vi "OpenNewFile.vi"(8 "error in (no error)":errorcluster, 10 "targetFolder":path, 11 "FileAppender in":refnum<class "FileAppender.lvclass">) -> (0 "error out":errorcluster, 3 "FileAppender out":refnum<class "FileAppender.lvclass">)   [LabVIEW 2026, in "Lumberjack.lvlib" / "FileAppender.lvclass"]
uses:
  FileAppender.lvclass
  FileAppender.lvclass/FileAppender.ctl
  Lumberjack.lvlib
  Appender.lvclass/Appender.lvclass
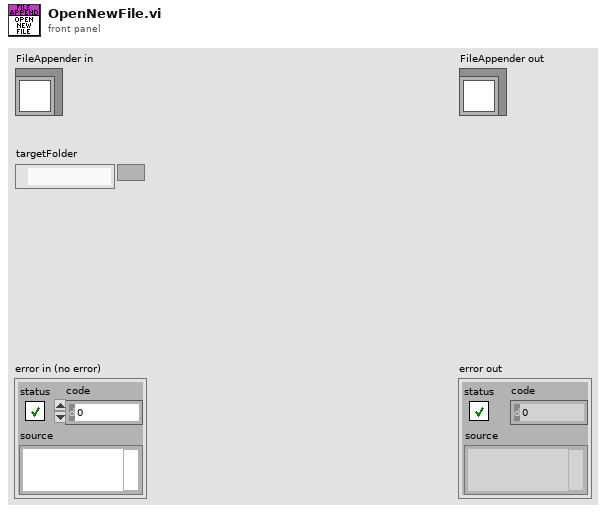
[diagram p1: front panel]
types:
  T1 = enum16{"open", "replace", "create", "open or create", "replace or create", "replace or create with confirmation"}
  T2 = typedef "Lumberjack.lvlib/AppenderConfig.ctl" = cluster{"id":string, "threshold":T3, "filter":T4, "queueBound":i32, "dropPolicy":T6, "useUTC":bool}
  T3 = typedef "Lumberjack.lvlib/Severity.ctl" = enum16{"OFF", "FATAL", "ERROR", "WARN", "INFO", "DEBUG", "TRACE", "ALL"}
  T4 = typedef "Lumberjack.lvlib/Filter.ctl" = cluster{"mode":T5, "levelMin":T3, "levelMax":T3, "tagPrefix":string}
  T5 = typedef "Lumberjack.lvlib/FilterMode.ctl" = enum16{"Mirror", "Routed"}
  T6 = typedef "Lumberjack.lvlib/DropPolicy.ctl" = enum16{"DropOldest", "DropNewest", "LevelAware"}
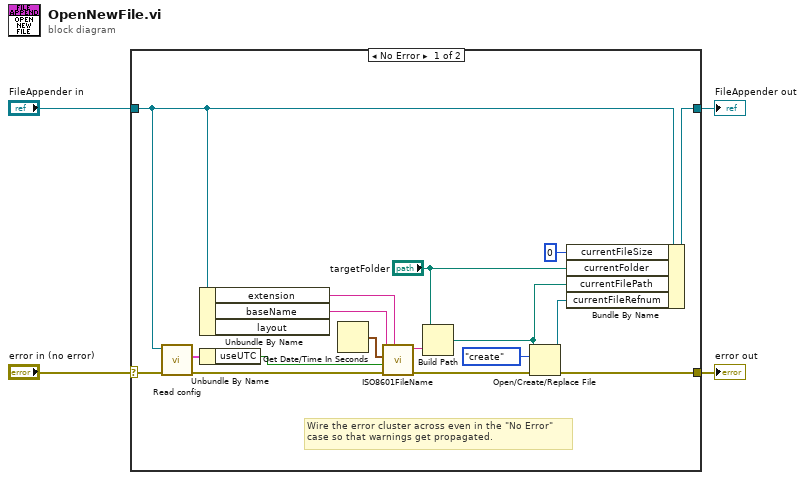
[diagram p0: block diagram]
diagram:
  n1 = case shown="No Error" "error in (no error)" {
    selector: "error in (no error)" -> [w15 w23]
    tunnel: [w20 w23] -> w3
    tunnel: [w21 w22] -> w1
    tunnel: "FileAppender in" -> [w14 w22]
    frame No Error {
      # "Wire the error cluster across even in the \"No Error\"\ncase so that warnings get propagated."
      n2 = call "Read config.vi"("error in (no error)"=w15, "Appender in"=w14) -> ("error out"=w13:errorcluster, "AppenderConfig"=w12:T2)  [unwired: 7 in, 1 out]
      n3 = Unbundle By Name(w14) -> ("extension"=w16:string, "baseName"=w17:string)  [unwired: 1 out]
      n4 = Unbundle By Name(w12) -> ("useUTC"=w11:bool)
      n5 = Get Date/Time In Seconds() -> (seconds since 1Jan1904=w18:timestamp)
      n6 = call "ISO8601FileName.vi"("Extension"=w16, "error in (no error)"=w13, "useUTC"=w11, "Timestamp"=w18, "BaseName"=w17) -> ("error out"=w19:errorcluster, "FileName"=w8:string)  [unwired: 5 in]
      n7 = Build Path(base path="targetFolder", name or relative path=w8) -> (appended path=w5:path)
      n8 = Open/Create/Replace File(file path (use dialog)=w5, error in=w19, operation (0:open)=T1."create") -> (refnum out=w6:refnum<file>, error out=w20:errorcluster)  [unwired: 3 in, 1 out]
      n9 = Bundle By Name(cluster=w14, "currentFileSize"=i64 0, "currentFolder"="targetFolder", "currentFilePath"=w5, "currentFileRefnum"=w6) -> (w21:refnum<class "FileAppender.lvclass">)
    }
    frame Error {
    }
  }
  "error out" <- w3
  "FileAppender out" <- w1
